vi "Bulk Add DI Coil - Right Click.vi"(11 "Node Ptr":T1 format="%.0x") -> ()   [LabVIEW 2015, in "Modbus Master System Explorer.lvlib"]
uses:
  <vilib>/NI Veristand/Custom Device API/Custom Device Item Ref.ctl
  Modbus Type.ctl
  Modbus Master System Explorer.lvlib
  <vilib>/NI VeriStand/Custom Device API/Custom Device API.lvlib
  Shared/Modbus Master Shared.lvlib
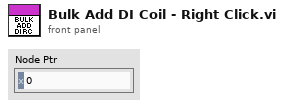
[diagram p1: front panel]
types:
  T1 = typedef "Custom Device API.lvlib/Custom Device Item Ref.ctl" = u64
  T2 = typedef "Modbus Master Shared.lvlib/Modbus Type.ctl" = enum16{"Coil", "Discrete Input", "Holding Register", "Input Register"}
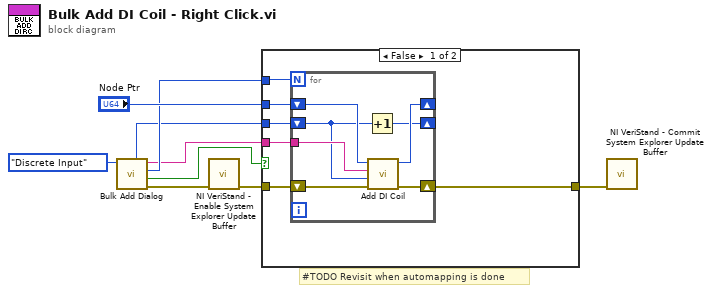
[diagram p0: block diagram]
diagram:
  # "#TODO Revisit when automapping is done"
  n1 = call "Bulk Add Dialog.vi"("Type"=Modbus_Type."Discrete Input") -> ("error out"=w4:errorcluster, "Cancelled?"=w7:bool, "Quantity Out"=w8:u16, "Root Name Out"=w6:string, "Starting Address Out"=w5:u16)  [unwired: 4 in, 2 out]
  n2 = call <vilib>:"NI VeriStand - Enable System Explorer Update Buffer.vi"("error in (no error)"=w4) -> ("error out"=w3:errorcluster)  [unwired: 10 in]
  n3 = case shown="False" w7 {
    tunnel: "Node Ptr" -> [w15 _]
    tunnel: w8 -> [w14 _]
    tunnel: w3 -> [w13 w23]
    tunnel: w6 -> [w12 _]
    tunnel: w5 -> [w11 _]
    tunnel: [w10 w23] -> w2
    frame False {
      n4 = for {
        N: w14 -> [_]
        shift-right: [w20] -> _
        shift-left: w15 -> [w22]
        shift-right: [w17] -> w10
        shift-left: w13 -> [w21]
        tunnel: w12 -> [w18]
        shift-right: [w19] -> _
        shift-left: w11 -> [w16]
        n5 = Increment(x=w16) -> (x+1=w19:u16)
        n6 = call "Add DI Coil.vi"("error in (no error)"=w21, "Starting Address"=w16, "Label"=w18, "Node Ref In"=w22) -> ("error out"=w17:errorcluster, "Node Ref out"=w20:T1)  [unwired: 5 in, 1 out]
      }
    }
    frame True {
    }
  }
  n7 = call <vilib>:"NI VeriStand - Commit System Explorer Update Buffer.vi"("error in (no error)"=w2) -> ()  [unwired: 10 in, 1 out]
